vi "Teleop.vi"(10 "Match Info":T1={"Autonomous Elapsed Seconds"=0.0, "TeleOp Elapsed Seconds"=0.0, "Disabled Elapsed Seconds"=0.0, "Visited Autonomous"=FALSE, "Visited TeleOp"=FALSE, "Visited Disabled"=FALSE, "Autonomous Settings"={"Autonomous Style"=enum."Independent", "VI Refnum"=refnum}}, 11 "Call Context":T2) -> ()   [LabVIEW 2019]
doc: "This VI is called for each TeleOp packet received from the DS where the robot is not disabled. It is often used to read from the joysticks and update I/O or to update setpoints for timed control loops. It should complete and return within 20 milliseconds or it may miss DS packets."
uses:
  <vilib>/Rock Robotics/WPI/DriverStation/WPI_DriverStationDerivedRobotMode.ctl
  <vilib>/Rock Robotics/WPI/DriverStation/WPI_DriverStationMatch Info.ctl
  <vilib>/Rock Robotics/WPI/Utilities/WPI_GetSetVariantRefNum.vi
  Robot Global Data.vi
  <vilib>/Rock Robotics/Network Tables/NT Write Number.vi
  <vilib>/Rock Robotics/Network Tables/NT Write Boolean.vi
panel:
  # "Click here to set min"
  # "Click here to set max"
  # "Click here to set min"
  # "Click here to set max"
  # "Click here to set min"
  # "Click here to set max"
  # "Click here to set min"
  # "Click here to set max"
  # "Click here to set min"
  # "Click here to set max"
  # "Click here to set min"
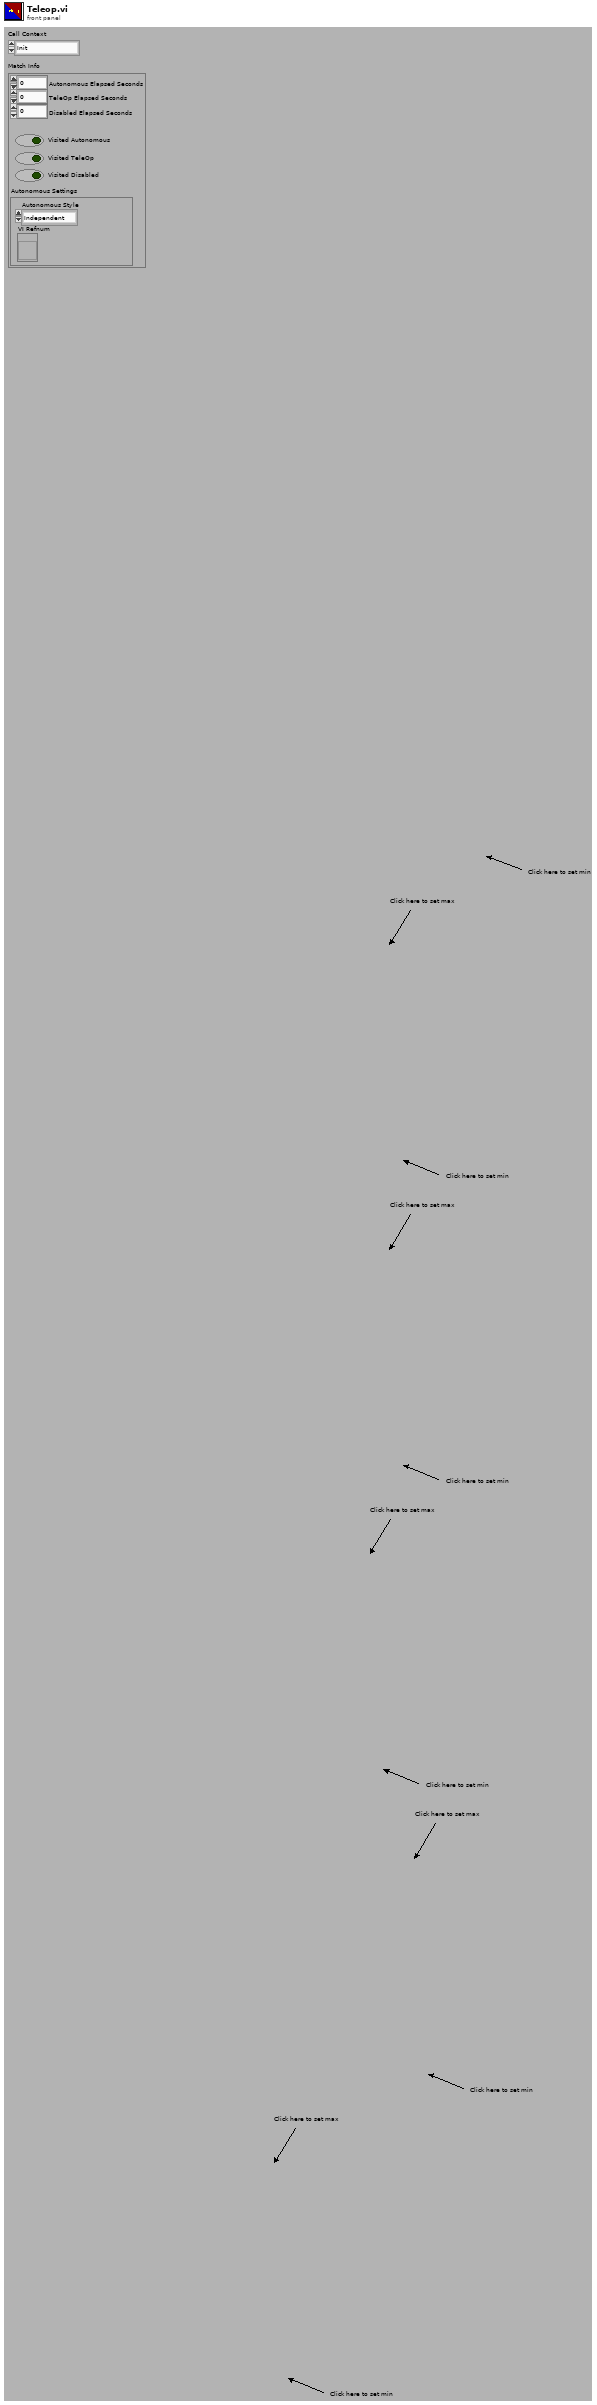
[diagram p1: front panel]
types:
  T1 = typedef "WPI_DriverStationMatch Info.ctl" = cluster{"Autonomous Elapsed Seconds":dbl, "TeleOp Elapsed Seconds":dbl, "Disabled Elapsed Seconds":dbl, "Visited Autonomous":bool, "Visited TeleOp":bool, "Visited Disabled":bool, "Autonomous Settings":cluster{"Autonomous Style":enum16{"Iterative", "Independent"}, "VI Refnum":refnum<vi>}}
  T2 = typedef "WPI_DriverStationDerivedRobotMode.ctl" = enum16{"Init", "Execute", "Stop"}
  T3 = typedef "WPI_JoystickDevRef.ctl" = cluster{"Device":T4}
  T4 = typedef "WPI_JoystickDeviceEnum.ctl" = enum16{"USB 0", "USB 1", "USB 2", "USB 3", "USB 4", "USB 5"}
  T5 = typedef "WPI_RobotDriveDevRef.ctl" = cluster{"DevStatus":errorcluster, "Motors[]":T6[], "Square Inputs":bool, "Max Output":dbl}
  T6 = typedef "WPI_MotorControlDeviceRef.ctl" = cluster{"DeviceStatus":errorcluster, "Type":T7, "PWM":cluster{"PWM Channel":T8, "DeadBand":T9}, "CAN":cluster{"Device Number":u8, "SetOutput VI Ref":variant, "GetOutput VI Ref":variant, "Enable VI Ref":variant, "Disable VI Ref":variant, "Data":variant}, "Invert":bool, "DIO PWM":cluster{"PWM \"Enable\" Channel":T8, "DIOChannel":T10, "PWM Rate":dbl}}
  T7 = typedef "WPI_MotorControlType.ctl" = enum16{"PWM", "CAN", "DIO PWM"}
  T8 = typedef "FPGA_DIOPWMChannel.ctl" = enum8{"PWM 0", "PWM 1", "PWM 2", "PWM 3", "PWM 4", "PWM 5", "PWM 6", "PWM 7", "PWM 8", "PWM 9", "PWM MXP 0", "PWM MXP 1", "PWM MXP 2", "PWM MXP 3", "PWM MXP 4", "PWM MXP 5", "PWM MXP 6", "PWM MXP 7", "PWM MXP 8", "PWM MXP 9", "Invalid"}
  T9 = typedef "WPI_PWMDeadband.ctl" = cluster{"Name":string, "maxPositivePwm":i32, "minPositivePwm":i32, "centerPwm":i32, "maxNegativePwm":i32, "minNegativePwm":i32, "angularRange":u16}
  T10 = typedef "FPGA_DIOChannel.ctl" = enum8{"DIO 0", "DIO 1", "DIO 2", "DIO 3", "DIO 4", "DIO 5", "DIO 6", "DIO 7", "DIO 8", "DIO 9", "DIO MXP 0", "DIO MXP 1", "DIO MXP 2", "DIO MXP 3", "DIO MXP 4", "DIO MXP 5", "DIO MXP 6", "DIO MXP 7", "DIO MXP 8", "DIO MXP 9", "DIO MXP 10", "DIO MXP 11", "DIO MXP 12", "DIO MXP 13", "DIO MXP 14", "DIO MXP 15", "SPI Port CS1", "SPI Port CS2", "SPI Port CS3", "SPI Port MISO", "SPI Port MOSI", "Invalid"}
  T11 = cluster{"JoystickDevRef":T3, "RobotDriveDevRef":T5}
  T12 = typedef "WPI_ServoDeviceRef.ctl" = cluster{"DeviceStatus":errorcluster, "PWM Channel":T8, "DeadBand":T9}
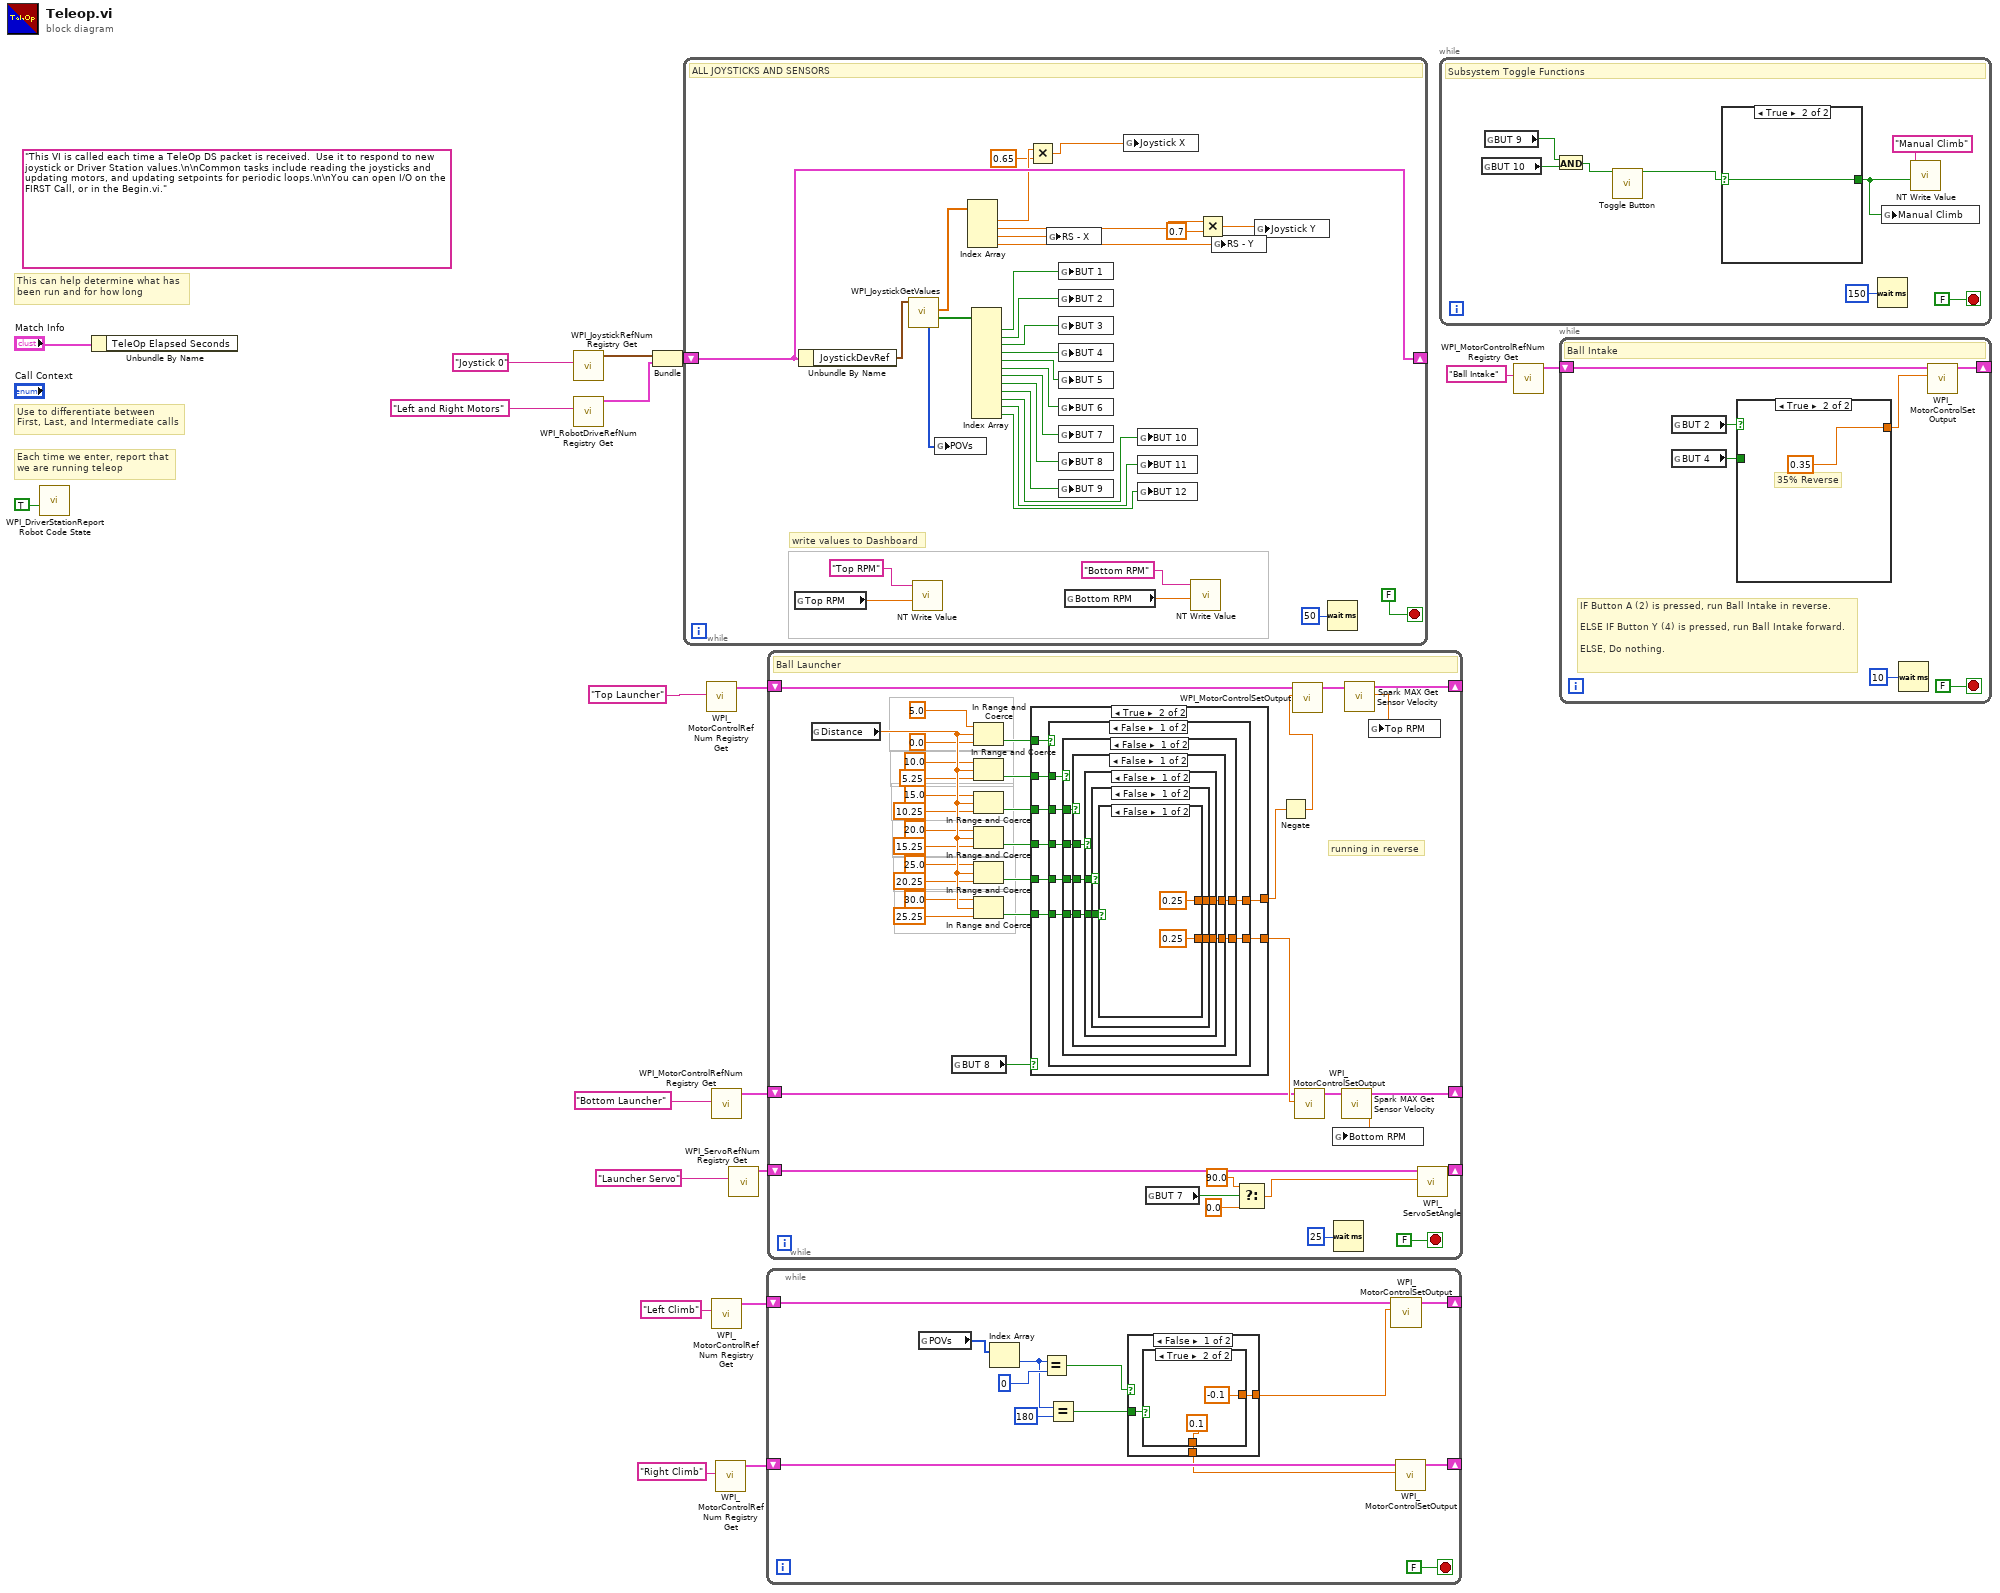
[diagram p0: block diagram]
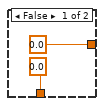
[diagram p2: hidden frame]
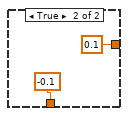
[diagram p3: hidden frame]
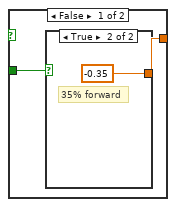
[diagram p4: hidden frame]
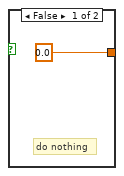
[diagram p5: hidden frame]
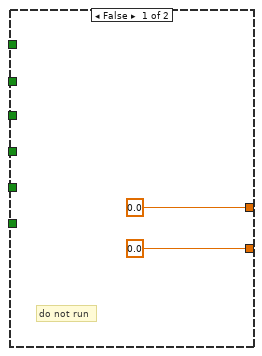
[diagram p7: hidden frame]
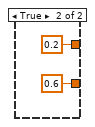
[diagram p8: hidden frame]
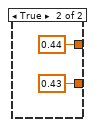
[diagram p9: hidden frame]
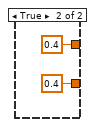
[diagram p10: hidden frame]
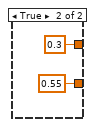
[diagram p11: hidden frame]
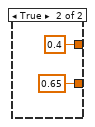
[diagram p12: hidden frame]
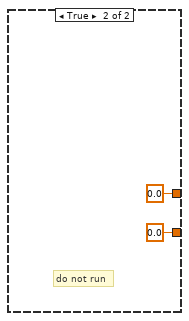
[diagram p13: hidden frame]
diagram:
  (unwired) "This VI is called each time a TeleOp DS packet is received.  Use it to respond to new joystick or Driver Station values.\n\nCommon tasks include reading the joysticks and updating motors, and updating setpoints for periodic loops.\n\nYou can open I/O on the FIRST Call, or in the Begin.vi."
  # "Each time we enter, report that\nwe are running teleop"
  # "Use to differentiate between\nFirst, Last, and Intermediate calls"
  # "This can help determine what has\nbeen run and for how long"
  n1 = call <vilib>:"WPI_DriverStationReport Robot Code State.vi"("TeleOp"=TRUE ("Autonomous")) -> ()  [unwired: 10 in, 1 out]
  n2 = Unbundle By Name("Match Info") -> ()  [unwired: 1 out]
  n3 = call <vilib>:"WPI_JoystickRefNum Registry Get.vi"("refnum name"="Joystick 0") -> ("JoystickDevRef"=w15:T3)  [unwired: 1 in, 9 out]
  n4 = call <vilib>:"WPI_RobotDriveRefNum Registry Get.vi"("refnum name"="Left and Right Motors") -> ("RobotDriveDevRef"=w14:T5)  [unwired: 1 in, 9 out]
  n5 = Bundle("JoystickDevRef"=w15, "RobotDriveDevRef"=w14) -> (w13:T11)  [unwired: 1 out]
  n6 = while {
    shift-right: [w35] -> _
    shift-left: w13 -> [w35]
    stop <- FALSE stop-if-true
    # "write values to Dashboard"
    # "ALL JOYSTICKS AND SENSORS"
    n7 = global read "Robot Global Data.vi" "Top RPM"() -> (w30:dbl)
    n8 = Unbundle By Name(w35) -> ("JoystickDevRef"=w49:T3)
    n9 = call <vilib>:"WPI_JoystickGetValues.vi"("JoystickDevRef"=w49) -> ("Buttons"=w48:bool[], "Axes"=w34:dbl[], "POVs"=w26:i16[])  [unwired: 6 in, 2 out]
    n10 = call-poly <vilib>:"NT Write Value.vi"("Numeric"=w30, "Name"="Top RPM") -> ()  [unwired: 9 in, 1 out]
    n11 = global write "Robot Global Data.vi" "POVs"(w26) -> ()
    n12 = Index Array(array=w34) -> (element #1=w23:dbl, element #2=w25:dbl, element #3=w27:dbl, element #4=w33:dbl)  [unwired: 4 in]
    n13 = Index Array(array=w48) -> (element #1=w47:bool, element #2=w46:bool, element #3=w45:bool, element #4=w44:bool, element #5=w43:bool, element #6=w42:bool, element #7=w41:bool, element #8=w40:bool, element #9=w39:bool, element #10=w38:bool, element #11=w37:bool, element #12=w36:bool)  [unwired: 12 in]
    n14 = Multiply(x=w23, y=0.65) -> (x*y=w24:dbl)
    n15 = global write "Robot Global Data.vi" "RS - X"(w27) -> ()
    n16 = global write "Robot Global Data.vi" "BUT 1"(w47) -> ()
    n17 = global write "Robot Global Data.vi" "BUT 2"(w46) -> ()
    n18 = global write "Robot Global Data.vi" "BUT 3"(w45) -> ()
    n19 = global write "Robot Global Data.vi" "BUT 4"(w44) -> ()
    n20 = global write "Robot Global Data.vi" "BUT 5"(w43) -> ()
    n21 = global write "Robot Global Data.vi" "BUT 6"(w42) -> ()
    n22 = global write "Robot Global Data.vi" "BUT 7"(w41) -> ()
    n23 = global write "Robot Global Data.vi" "BUT 8"(w40) -> ()
    n24 = global write "Robot Global Data.vi" "BUT 9"(w39) -> ()
    n25 = global read "Robot Global Data.vi" "Bottom RPM"() -> (w28:dbl)
    n26 = global write "Robot Global Data.vi" "Joystick X"(w24) -> ()
    n27 = global write "Robot Global Data.vi" "BUT 10"(w38) -> ()
    n28 = global write "Robot Global Data.vi" "BUT 11"(w37) -> ()
    n29 = global write "Robot Global Data.vi" "BUT 12"(w36) -> ()
    n30 = call-poly <vilib>:"NT Write Value.vi"("Numeric"=w28, "Name"="Bottom RPM") -> ()  [unwired: 9 in, 1 out]
    n31 = Multiply(x=w25, y=0.7) -> (x*y=w21:dbl)
    n32 = global write "Robot Global Data.vi" "RS - Y"(w33) -> ()
    n33 = global write "Robot Global Data.vi" "Joystick Y"(w21) -> ()
    n34 = Wait (ms)(milliseconds to wait=u32 50) -> ()  [unwired: 1 out]
  }
  n35 = call <vilib>:"WPI_MotorControlRefNum Registry Get.vi"("refnum name"="Top Launcher") -> ("MotorControlDevRef"=w9:T6)  [unwired: 9 in, 1 out]
  n36 = call <vilib>:"WPI_MotorControlRefNum Registry Get.vi"("refnum name"="Bottom Launcher") -> ("MotorControlDevRef"=w11:T6)  [unwired: 9 in, 1 out]
  n37 = call <vilib>:"WPI_MotorControlRefNum Registry Get.vi"("refnum name"="Left Climb") -> ("MotorControlDevRef"=w3:T6)  [unwired: 9 in, 1 out]
  n38 = call <vilib>:"WPI_MotorControlRefNum Registry Get.vi"("refnum name"="Right Climb") -> ("MotorControlDevRef"=w2:T6)  [unwired: 9 in, 1 out]
  n39 = call <vilib>:"WPI_ServoRefNum Registry Get.vi"("refnum name"="Launcher Servo") -> ("ServoDeviceRef"=w7:T12)  [unwired: 9 in, 1 out]
  n40 = while {
    shift-right: [w62] -> _
    shift-left: w3 -> [w61]
    shift-right: [w59] -> _
    shift-left: w2 -> [w60]
    stop <- FALSE stop-if-true
    n41 = global read "Robot Global Data.vi" "POVs"() -> (w56:i16[])
    n42 = Index Array(array=w56) -> (element=w52:i16)  [unwired: 1 in]
    n43 = Equal?(x=w52, y=i16 0) -> (x = y?=w54:bool)
    n44 = Equal?(x=w52, y=i16 180) -> (x = y?=w53:bool)
    n45 = case shown="False" w54 {
      tunnel: [w66 0.1 ("Output")] -> w58
      tunnel: [w65 -0.1 ("Output")] -> w57
      tunnel: w53 -> [w64 _]
      frame False {
        n46 = case shown="True" w64 {
          tunnel: [0.0 ("Output") -0.1 ("Output")] -> w66
          tunnel: [0.0 ("Output") 0.1 ("Output")] -> w65
          frame False {
          }
          frame True {
          }
        }
      }
      frame True {
      }
    }
    n47 = call <vilib>:"WPI_MotorControlSetOutput.vi"("Output"=w58, "MotorControlDevRef"=w61) -> ("MotorControlDevRef"=w62:T6)  [unwired: 7 in, 2 out]
    n48 = call <vilib>:"WPI_MotorControlSetOutput.vi"("Output"=w57, "MotorControlDevRef"=w60) -> ("MotorControlDevRef"=w59:T6)  [unwired: 7 in, 2 out]
  }
  n49 = while {
    shift-right: [w81] -> _
    shift-left: w11 -> [w82]
    shift-right: [w79] -> _
    shift-left: w9 -> [w80]
    shift-right: [w78] -> _
    shift-left: w7 -> [w73]
    stop <- FALSE stop-if-true
    # "running in reverse"
    # "Ball Launcher"
    n50 = global read "Robot Global Data.vi" "Distance"() -> (w111:dbl)
    n51 = global read "Robot Global Data.vi" "BUT 8"() -> (w89:bool)
    n52 = In Range and Coerce(upper limit=5.0, x=w111, lower limit=0.0) -> (In Range?=w108:bool)  [unwired: 1 out]
    n53 = In Range and Coerce(upper limit=10.0, x=w111, lower limit=5.25) -> (In Range?=w107:bool)  [unwired: 1 out]
    n54 = In Range and Coerce(upper limit=15.0, x=w111, lower limit=10.25) -> (In Range?=w91:bool)  [unwired: 1 out]
    n55 = In Range and Coerce(upper limit=20.0, x=w111, lower limit=15.25) -> (In Range?=w92:bool)  [unwired: 1 out]
    n56 = In Range and Coerce(upper limit=25.0, x=w111, lower limit=20.25) -> (In Range?=w93:bool)  [unwired: 1 out]
    n57 = In Range and Coerce(upper limit=30.0, x=w111, lower limit=25.25) -> (In Range?=w94:bool)  [unwired: 1 out]
    n58 = case shown="True" w89 {
      tunnel: [0.0 ("Output") w115] -> w110
      tunnel: [0.0 ("Output") w114] -> w90
      tunnel: w108 -> [_ w121]
      tunnel: w91 -> [_ w119]
      tunnel: w92 -> [_ w118]
      tunnel: w93 -> [_ w117]
      tunnel: w94 -> [_ w116]
      tunnel: w107 -> [_ w120]
      frame False {
        # "do not run"
      }
      frame True {
        n59 = case shown="False" w121 {
          tunnel: w120 -> [w128 _]
          tunnel: w119 -> [w127 _]
          tunnel: w118 -> [w126 _]
          tunnel: w117 -> [w125 _]
          tunnel: w116 -> [w124 _]
          tunnel: [w123 0.0 ("Output")] -> w115
          tunnel: [w122 0.0 ("Output")] -> w114
          frame False {
            n60 = case shown="False" w128 {
              tunnel: w127 -> [w134 _]
              tunnel: w126 -> [w133 _]
              tunnel: w125 -> [w132 _]
              tunnel: w124 -> [w131 _]
              tunnel: [w130 0.4 ("Output")] -> w123
              tunnel: [w129 0.65 ("Output")] -> w122
              frame False {
                n61 = case shown="False" w134 {
                  tunnel: w133 -> [w139 _]
                  tunnel: w132 -> [w138 _]
                  tunnel: w131 -> [w137 _]
                  tunnel: [w136 0.3 ("Output")] -> w130
                  tunnel: [w135 0.55 ("Output")] -> w129
                  frame False {
                    n62 = case shown="False" w139 {
                      tunnel: w138 -> [w143 _]
                      tunnel: w137 -> [w142 _]
                      tunnel: [w141 0.4 ("Output")] -> w136
                      tunnel: [w140 0.4 ("Output")] -> w135
                      frame False {
                        n63 = case shown="False" w143 {
                          tunnel: w142 -> [w146 _]
                          tunnel: [w145 0.44 ("Output")] -> w141
                          tunnel: [w144 0.43 ("Output")] -> w140
                          frame False {
                            n64 = case shown="False" w146 {
                              tunnel: [0.25 ("Output") 0.2 ("Output")] -> w145
                              tunnel: [0.25 ("Output") 0.6 ("Output")] -> w144
                              frame False {
                              }
                              frame True {
                              }
                            }
                          }
                          frame True {
                          }
                        }
                      }
                      frame True {
                      }
                    }
                  }
                  frame True {
                  }
                }
              }
              frame True {
              }
            }
          }
          frame True {
            # "do not run"
          }
        }
      }
    }
    n65 = global read "Robot Global Data.vi" "BUT 7"() -> (w77:bool)
    n66 = Select(t=90.0, s=w77, f=0.0) -> (s? t:f=w74:dbl)
    n67 = Negate(x=w110) -> (-x=w109:dbl)
    n68 = call <vilib>:"WPI_MotorControlSetOutput.vi"("Output"=w109, "MotorControlDevRef"=w80) -> ("MotorControlDevRef"=w87:T6)  [unwired: 7 in, 2 out]
    n69 = call <vilib>:"WPI_MotorControlSetOutput.vi"("Output"=w90, "MotorControlDevRef"=w82) -> ("MotorControlDevRef"=w88:T6)  [unwired: 7 in, 2 out]
    n70 = Wait (ms)(milliseconds to wait=u32 25) -> ()  [unwired: 1 out]
    n71 = call <vilib>:"Spark MAX Get Sensor Velocity.vi"("MotorControlDevRef in"=w88) -> ("Sensor Velocity"=w86:dbl, "MotorControlDevRef out"=w81:T6)  [unwired: 7 in, 2 out]
    n72 = global write "Robot Global Data.vi" "Bottom RPM"(w86) -> ()
    n73 = call <vilib>:"Spark MAX Get Sensor Velocity.vi"("MotorControlDevRef in"=w87) -> ("Sensor Velocity"=w85:dbl, "MotorControlDevRef out"=w79:T6)  [unwired: 7 in, 2 out]
    n74 = global write "Robot Global Data.vi" "Top RPM"(w85) -> ()
    n75 = call <vilib>:"WPI_ServoSetAngle.vi"("Angle"=w74, "ServoDeviceRef"=w73) -> ("ServoDeviceRef"=w78:T12)  [unwired: 8 in, 1 out]
  }
  n76 = while {
    stop <- FALSE stop-if-true
    # "Subsystem Toggle Functions"
    n77 = global read "Robot Global Data.vi" "BUT 10"() -> (w164:bool)
    n78 = global read "Robot Global Data.vi" "BUT 9"() -> (w166:bool)
    n79 = And(x=w166, y=w164) -> (x .and. y?=w165:bool)
    n80 = call "Toggle Button.vi"("Boolean in"=w165) -> ("Boolean out"=w163:bool)  [unwired: 10 in]
    n81 = case shown="True" w163 {
      selector: w163 -> [w169 w170]
      tunnel: [w169 w170] -> w162
      frame False {
      }
      frame True {
      }
    }
    n82 = Wait (ms)(milliseconds to wait=u32 150) -> ()  [unwired: 1 out]
    n83 = global write "Robot Global Data.vi" "Manual Climb"(w162) -> ()
    n84 = call-poly <vilib>:"NT Write Value.vi"("Boolean"=w162, "Name"="Manual Climb") -> ()  [unwired: 9 in, 1 out]
  }
  n85 = call <vilib>:"WPI_MotorControlRefNum Registry Get.vi"("refnum name"="Ball Intake") -> ("MotorControlDevRef"=w5:T6)  [unwired: 9 in, 1 out]
  n86 = while {
    shift-right: [w174] -> _
    shift-left: w5 -> [w175]
    stop <- FALSE stop-if-true
    # "IF Button A (2) is pressed, run Ball Intake in reverse. \n\nELSE IF Button Y (4) is pressed, run Ball Intake forward.\n\nELSE, Do nothing."
    # "Ball Intake"
    n87 = global read "Robot Global Data.vi" "BUT 2"() -> (w172:bool)
    n88 = global read "Robot Global Data.vi" "BUT 4"() -> (w173:bool)
    n89 = case shown="True" w172 {
      tunnel: [w179 0.35 ("Output")] -> w171
      tunnel: w173 -> [w178 _]
      frame False {
        n90 = case shown="True" w178 {
          tunnel: [0.0 ("Output") -0.35 ("Output")] -> w179
          frame False {
            # "do nothing"
          }
          frame True {
            # "35% forward"
          }
        }
      }
      frame True {
        # "35% Reverse"
      }
    }
    n91 = Wait (ms)(milliseconds to wait=u32 10) -> ()  [unwired: 1 out]
    n92 = call <vilib>:"WPI_MotorControlSetOutput.vi"("Output"=w171, "MotorControlDevRef"=w175) -> ("MotorControlDevRef"=w174:T6)  [unwired: 7 in, 2 out]
  }
